vi "Reload Config.vi"(8 "error in (no error)":errorcluster, 11 "VolatusAPI in":refnum<class "VolatusAPI.lvclass">) -> (0 "error out":errorcluster, 3 "VolatusAPI out":refnum<class "VolatusAPI.lvclass">)   [LabVIEW 2020, in "Volatus.lvlib" / "VolatusAPI.lvclass"]
uses:
  VolatusAPI.lvclass
  VolatusAPI.lvclass/VolatusAPI.ctl
  System Config Identity/System Config Identity.lvclass
  MessageQ/MessageQ.lvclass
  C:/dev/lv20CE/relink/lv-volatus/Volatus/System Config Identity/System Config Identity.lvclass
  C:/dev/lv20CE/relink/lv-volatus/Volatus/Identity/Identity.lvclass
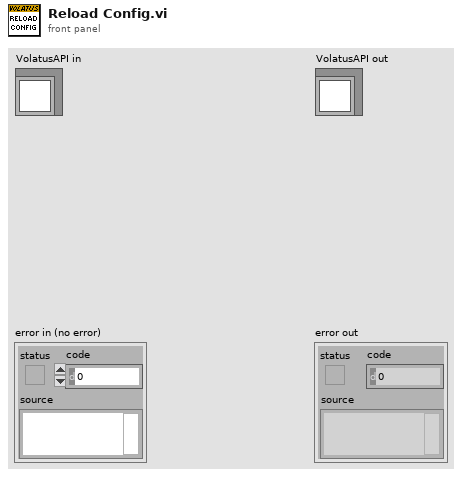
[diagram p1: front panel]
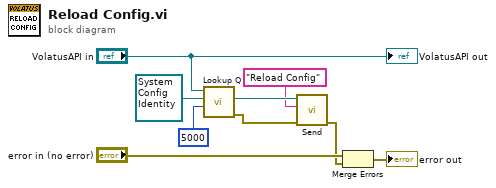
[diagram p0: block diagram]
diagram:
  n1 = call "Lookup Q.vi"("Timeout ms (0)"=5000, "Identity"=refnum<class "System Config Identity.lvclass"> refnum ("Volatus:System Config Identity.lvclass"), "VolatusAPI in"="VolatusAPI in") -> ("error out"=w4:errorcluster, "MessageQ"=w5:refnum<class "MessageQ.lvclass">)  [unwired: 6 in, 1 out]
  n2 = call "Send.vi"("error in (no error)"=w4, "ID"="Reload Config" ("Message ID"), "MessageQ in"=w5) -> ("error out"=w1:errorcluster)  [unwired: 7 in, 1 out]
  n3 = Merge Errors("error in (no error)", w1) -> (→"error out":errorcluster)
  "VolatusAPI out" <- "VolatusAPI in"
